vi "Logon - Module.vi"(6 "Main Application Directory":path, 7 "Logon - Enum":T2=enum."Check AD", 8 "Error In":errorcluster, 9 "Password":string, 10 "Domain":string, 11 "Logon User":string) -> (0 "Error Out":errorcluster, 1 "PC username Info":string[][](array[string]), 2 "Logon OK":bool, 3 "AD Info":T1, 4 "Hostname":string, 5 "standard output":string)   [LabVIEW 2013]
uses:
  Controls/Logon - Enum.ctl
  <vilib>/Utility/miscctls.llb/LVComboBoxStrsAndValuesArrayTypeDef.ctl
  <vilib>/Utility/error.llb/whitespace.ctl
panel:
  out "ERROR":string
  out "Full Name":string
  # "The request will be processed at a domain controller for domain ccc.coopcam.com."
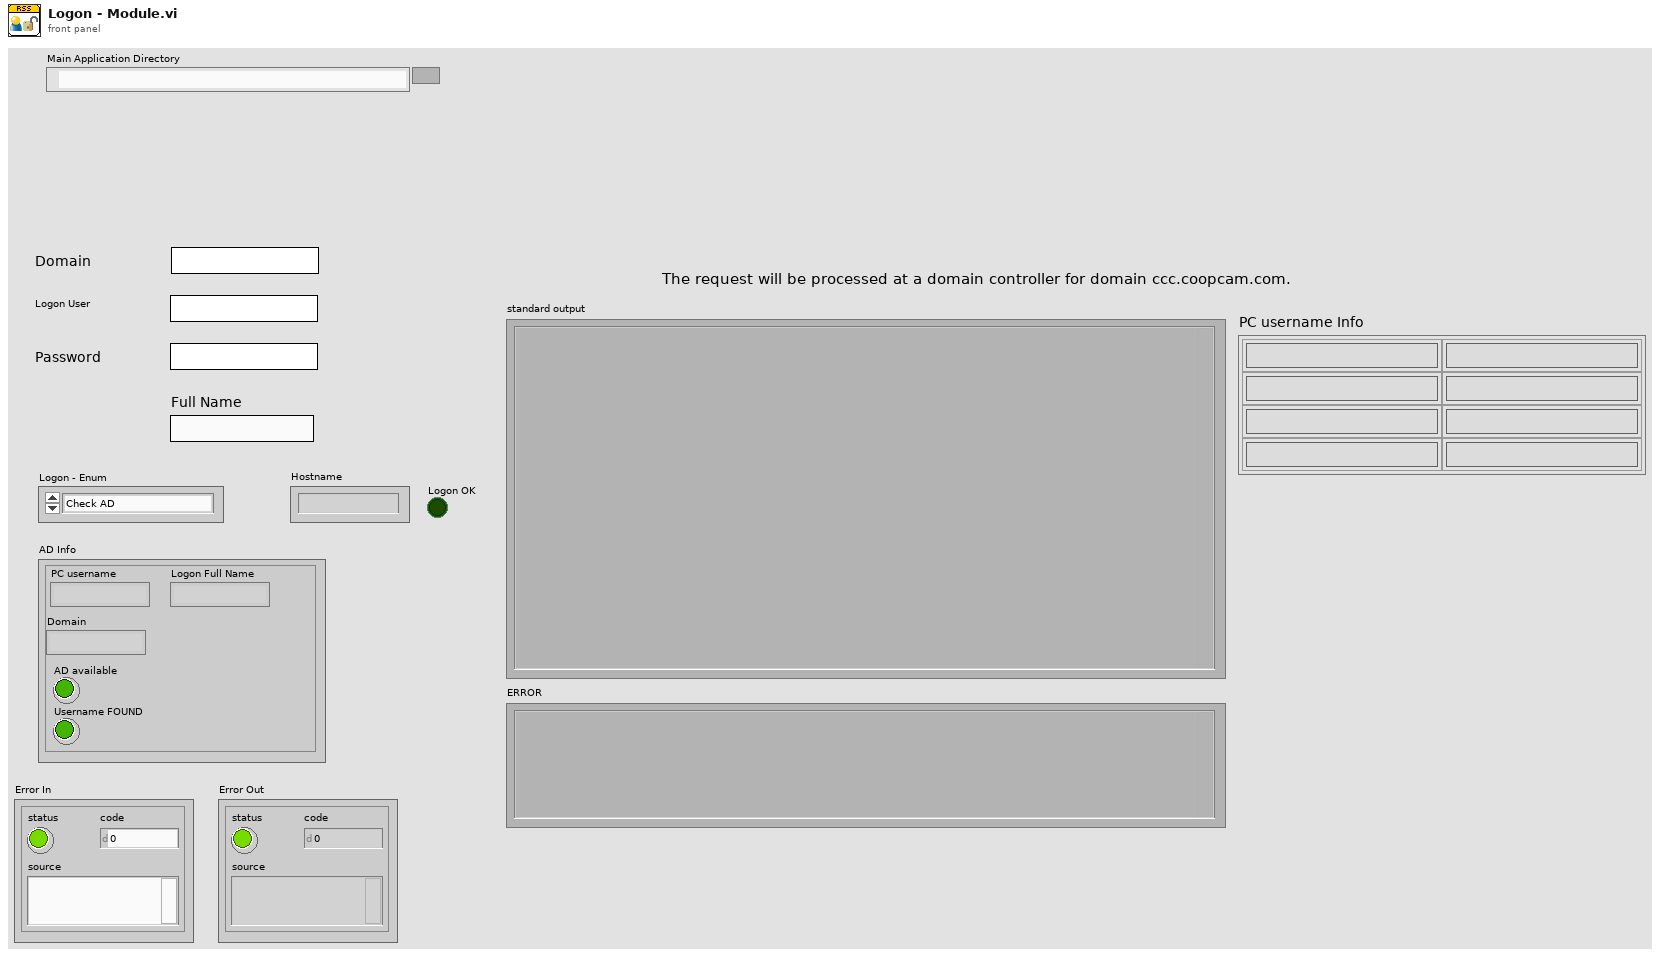
[diagram p1: front panel]
types:
  T1 = cluster{"PC username":string, "Domain":string, "AD available":bool, "Username FOUND":bool, "Logon Full Name":string}
  T2 = typedef "Logon - Enum.ctl" = enum16{"PC username", "PC username INFO", "Hostname", "Check AD", "Logon", "QUIT"}
  T3 = typedef "LVComboBoxStrsAndValuesArrayTypeDef.ctl" = cluster{"String":string, "Value":string}[]
  T4 = typedef "whitespace.ctl" = u16
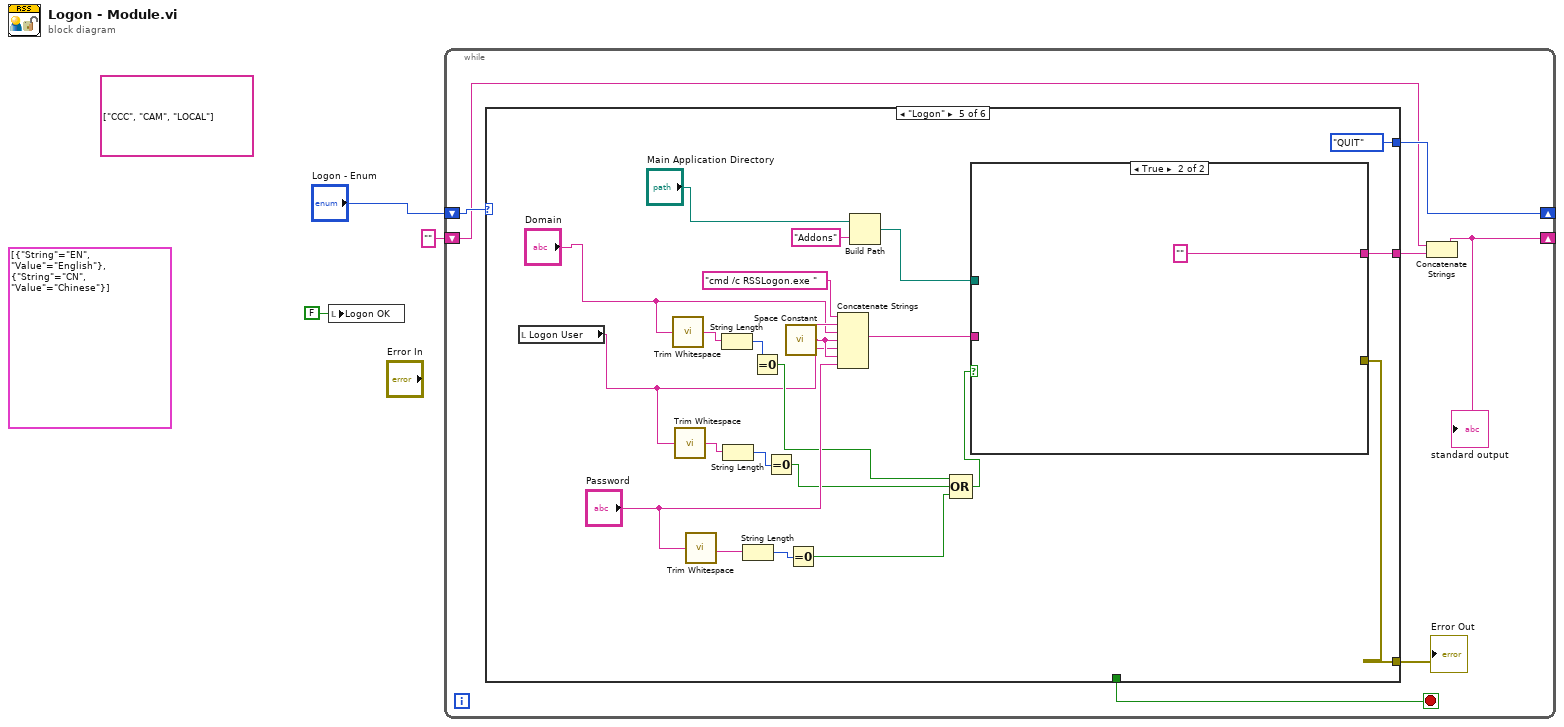
[diagram p0: block diagram]
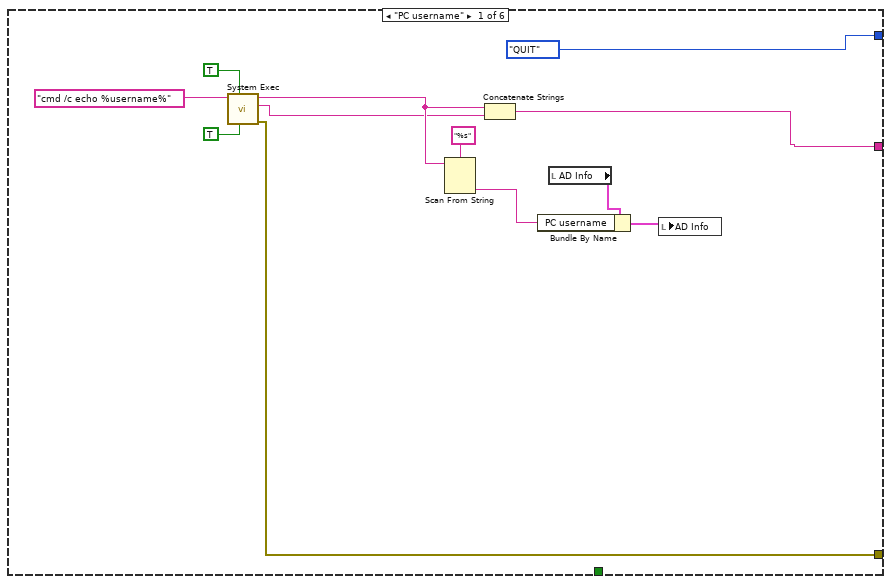
[diagram p2: hidden frame]
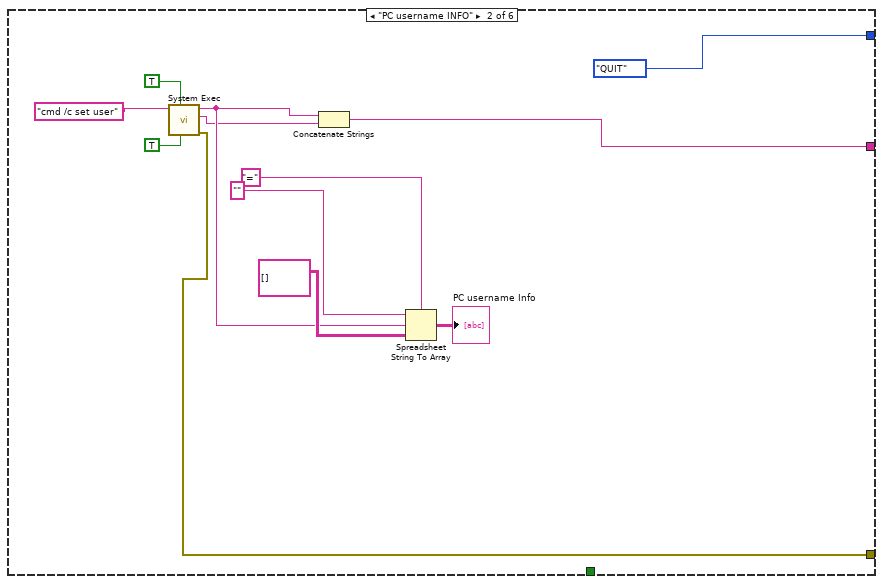
[diagram p3: hidden frame]
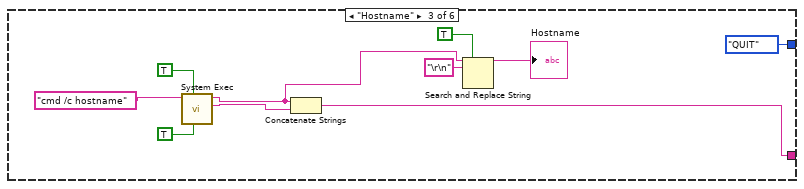
[diagram p4: hidden frame]
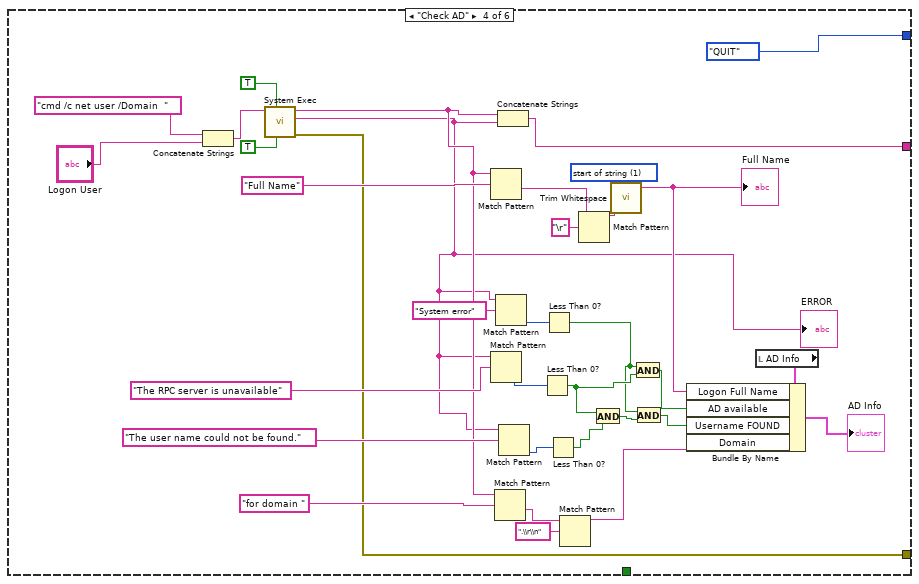
[diagram p5: hidden frame]
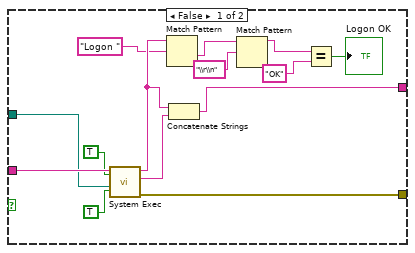
[diagram p6: hidden frame]
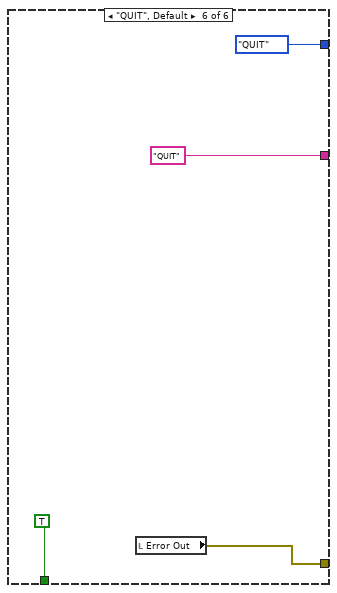
[diagram p7: hidden frame]
diagram:
  (unwired) T3 [{"String"="EN", "Value"="English"}, {"String"="CN", "Value"="Chinese"}] ("Strings And Values []")
  (unwired) string[] ["CCC", "CAM", "LOCAL"] ("Strings []")
  n1 = local write "Logon OK"(FALSE ("Logon OK")) -> ()
  n2 = while {
    shift-right: [w8] -> _
    shift-left: "Logon - Enum" -> [w10]
    shift-right: [w7] -> _
    shift-left: "" -> [w6]
    stop <- w9 stop-if-true
    n3 = case shown="\"Logon\"" w10 {
      tunnel: [_ _ _ _ _ TRUE] -> w9
      tunnel: [Logon_-_Enum."QUIT" ("Logon - Enum") Logon_-_Enum."QUIT" ("Logon - Enum") Logon_-_Enum."QUIT" ("Logon - Enum") Logon_-_Enum."QUIT" ("Logon - Enum") Logon_-_Enum."QUIT" ("Logon - Enum") Logon_-_Enum."QUIT" ("Logon - Enum")] -> w8
      tunnel: [w14 w23 w40 w57 w86 "QUIT" ("standard output")] -> w5
      tunnel: [w17 w26 _ w59 w85 w116] -> w4
      frame "PC username" {
        n4 = call <vilib>:"System Exec.vi"("run minimized? (F)"=TRUE, "wait until completion? (T)"=TRUE, "command line"="cmd /c echo %username%") -> ("error out"=w17:errorcluster, "standard error"=w15:string, "standard output"=w16:string)  [unwired: 5 in, 1 out]
        n5 = Scan From String(format string="%s", input string=w16) -> (output 1=w11:string)  [unwired: 3 in, 3 out]
        n6 = Concatenate Strings(w16, w15) -> (w14:string)
        n7 = local read "AD Info"() -> (w13:T1)
        n8 = Bundle By Name(cluster=w13, "PC username"=w11) -> (w12:T1)
        n9 = local write "AD Info"(w12) -> ()
      }
      frame "PC username INFO" {
        n10 = call <vilib>:"System Exec.vi"("run minimized? (F)"=TRUE, "wait until completion? (T)"=TRUE, "command line"="cmd /c set user") -> ("error out"=w26:errorcluster, "standard error"=w24:string, "standard output"=w25:string)  [unwired: 5 in, 1 out]
        n11 = Concatenate Strings(w25, w24) -> (w23:string)
        n12 = Spreadsheet String To Array(delimiter (Tab)="=", format string="", spreadsheet string=w25, array type (2D Dbl)=string[][] []) -> (array=→"PC username Info":string[][])
      }
      frame "Hostname" {
        n13 = call <vilib>:"System Exec.vi"("run minimized? (F)"=TRUE, "wait until completion? (T)"=TRUE, "command line"="cmd /c hostname") -> ("standard error"=w41:string, "standard output"=w38:string)  [unwired: 5 in, 2 out]
        n14 = Concatenate Strings(w38, w41) -> (w40:string)
        n15 = Search and Replace String(replace all?=TRUE ("replace all? (F)"), input string=w38, search string="\r\n") -> (result string=→"Hostname":string)  [unwired: 5 in, 3 out]
      }
      frame "Check AD" {
        w70 = T4 1 items=["both", "start of string", "end of string"] ("location (both)")
        n16 = Concatenate Strings("cmd /c net user /Domain  " ("command line"), "Logon User") -> (w75:string)
        n17 = call <vilib>:"System Exec.vi"("run minimized? (F)"=TRUE, "wait until completion? (T)"=TRUE, "command line"=w75) -> ("error out"=w59:errorcluster, "standard error"=w52:string, "standard output"=w58:string)  [unwired: 5 in, 1 out]
        "ERROR" <- w52
        n18 = Match Pattern(string=w58, regular expression="Full Name") -> (after substring=w73:string)  [unwired: 1 in, 3 out]
        n19 = Match Pattern(string=w52, regular expression="The RPC server is unavailable") -> (offset past match=w68:i32)  [unwired: 1 in, 3 out]
        n20 = Match Pattern(string=w58, regular expression="for domain ") -> (after substring=w61:string)  [unwired: 1 in, 3 out]
        n21 = Match Pattern(string=w52, regular expression="System error") -> (offset past match=w50:i32)  [unwired: 1 in, 3 out]
        n22 = Concatenate Strings(w58, w52) -> (w57:string)
        n23 = Match Pattern(string=w52, regular expression="The user name could not be found.") -> (offset past match=w65:i32)  [unwired: 1 in, 3 out]
        n24 = Less Than 0?(x=w68) -> (x < 0?=w49:bool)
        n25 = Less Than 0?(x=w50) -> (x < 0?=w47:bool)
        n26 = Less Than 0?(x=w65) -> (x < 0?=w64:bool)
        n27 = Match Pattern(string=w61, regular expression=".\\r\\n") -> (before substring=w55:string)  [unwired: 1 in, 3 out]
        n28 = Match Pattern(string=w73, regular expression="\r") -> (before substring=w71:string)  [unwired: 1 in, 3 out]
        n29 = And(x=w49, y=w64) -> (x .and. y?=w46:bool)
        n30 = call <vilib>:"Trim Whitespace.vi"("string"=w71, "location (both)"=w70) -> ("trimmed string"=w54:string)
        "Full Name" <- w54
        n31 = And(x=w47, y=w49) -> (x .and. y?=w48:bool)
        n32 = And(x=w47, y=w46) -> (x .and. y?=w45:bool)
        n33 = local read "AD Info"() -> (w56:T1)
        n34 = Bundle By Name(cluster=w56, "Logon Full Name"=w54, "AD available"=w48, "Username FOUND"=w45, "Domain"=w55) -> (→"AD Info":T1)
      }
      frame "Logon" {
        n35 = local read "Logon User"() -> (w84:string)
        n36 = call <vilib>:"Trim Whitespace.vi"("string"="Domain") -> ("trimmed string"=w96:string)  [unwired: 1 in]
        n37 = call <vilib>:"Trim Whitespace.vi"("string"=w84) -> ("trimmed string"=w95:string)  [unwired: 1 in]
        n38 = call <vilib>:"Trim Whitespace.vi"("string"="Password") -> ("trimmed string"=w94:string)  [unwired: 1 in]
        n39 = String Length(string=w96) -> (length=w93:i32)
        n40 = String Length(string=w95) -> (length=w92:i32)
        n41 = String Length(string=w94) -> (length=w91:i32)
        n42 = Equal To 0?(x=w93) -> (x = 0?=w90:bool)
        n43 = Equal To 0?(x=w92) -> (x = 0?=w89:bool)
        n44 = call <vilib>:"Space Constant.vi"() -> ("String"=w99:string)
        n45 = Equal To 0?(x=w91) -> (x = 0?=w88:bool)
        n46 = Concatenate Strings("cmd /c RSSLogon.exe " ("command line"), w99, "Domain", w99, w84, w99, "Password") -> (w100:string)
        n47 = Build Path(base path="Main Application Directory", name or relative path="Addons") -> (appended path=w80:path)
        n48 = Compound Arithmetic op=OR(w90, w89, w88) -> (w87:bool)
        n49 = case shown="True" w87 {
          tunnel: w100 -> [w114 _]
          tunnel: w80 -> [w111 _]
          tunnel: [w108 "" ("standard output")] -> w86
          tunnel: [w110 _] -> w85
          frame False {
            n50 = call <vilib>:"System Exec.vi"("run minimized? (F)"=TRUE, "wait until completion? (T)"=TRUE, "working directory"=w111, "command line"=w114) -> ("error out"=w110:errorcluster, "standard error"=w109:string, "standard output"=w107:string)  [unwired: 4 in, 1 out]
            n51 = Match Pattern(string=w107, regular expression="Logon ") -> (after substring=w105:string)  [unwired: 1 in, 3 out]
            n52 = Concatenate Strings(w107, w109) -> (w108:string)
            n53 = Match Pattern(string=w105, regular expression="\\r\\n") -> (before substring=w103:string)  [unwired: 1 in, 3 out]
            n54 = Equal?(x=w103, y="OK") -> (x = y?=→"Logon OK":bool)
          }
          frame True {
          }
        }
      }
      frame "QUIT", Default {
        n55 = local read "Error Out"() -> (w116:errorcluster)
      }
    }
    "Error Out" <- w4
    n56 = Concatenate Strings(w6, w5) -> (w7:string)
    "standard output" <- w7
  }
